vi "FL Set Membership Function.vi"   [LabVIEW 2017, in "NI_Fuzzy_Logic_API.lvlib"]
doc: "Modifies the shape, color, or points of a membership function for a linguistic variable. You can modify a membership function from a fuzzy system or from an array of membership functions. The data type you wire to the <B>fuzzy system in</B> input determines the polymorphic instance to use."
uses:
  <vilib>/addons/Fuzzy Logic/NI_Fuzzy_Logic_API.lvlib
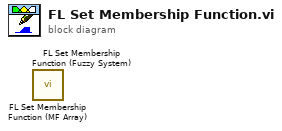
[diagram p0: block diagram]
diagram:
  n1 = call <vilib>:"FL Set Membership Function (MF Array).vi"() -> ()  [unwired: 14 in, 2 out]
  n2 = call <vilib>:"FL Set Membership Function (Fuzzy System).vi"() -> ()  [unwired: 14 in, 2 out]
